vi "Initialize JSON DAO.vi"(10 "Item Name":string="PA Order Tracker", 11 "DB Sufix":string) -> (0 "error out":errorcluster, 3 "Customer DAO JSON out":refnum<class "Object DAO JSON.lvclass">)   [LabVIEW 2020, in "Object DAO JSON.lvclass"]
uses:
  Object DAO JSON.lvclass
  C:/Users/fflores/Desktop/DataBase - Copy - Copy - Copy/Object DAO/Object DAO.lvclass
  Object DAO/Object DAO.lvclass/Object DAO.ctl
  Object DAO JSON.lvclass/Object DAO JSON.ctl
  Object DAO/Member Accessors/Get Item Name.vi
  External Libraries/JSON File Manipulation.lvlibp
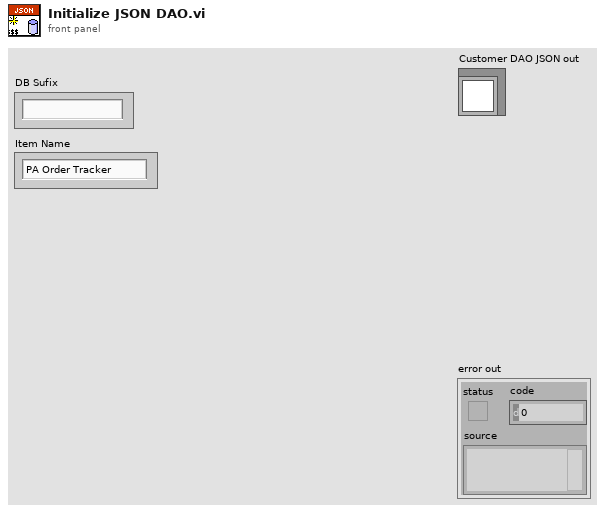
[diagram p1: front panel]
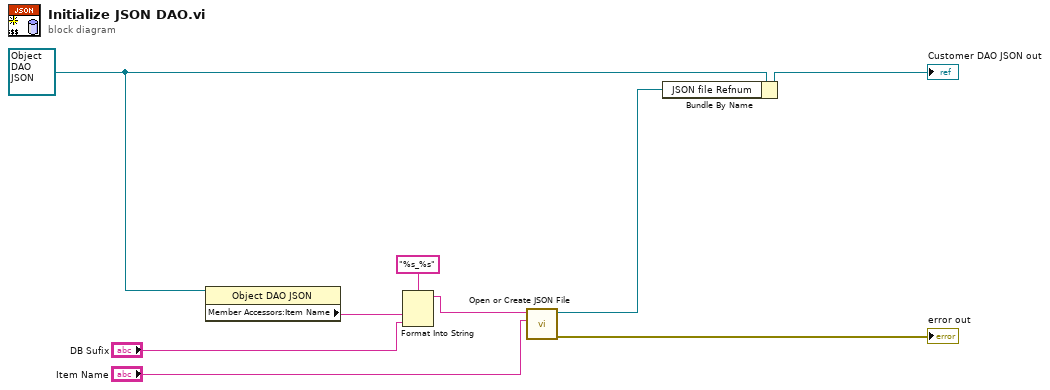
[diagram p0: block diagram]
diagram:
  w6 = refnum<class "Object DAO JSON.lvclass"> refnum ("Customer DAO JSON in")
  n1 = property class="Object DAO JSON"(reference=w6) -> ("Member Accessors:Item Name"=w5:string)  [unwired: 1 in, 2 out]
  n2 = Format Into String(format string="%s_%s", w5, "DB Sufix") -> (resulting string=w2:string)  [unwired: 2 in, 1 out]
  n3 = call "Open or Create JSON File.vi"("Application Name"="Item Name", "Item Name"=w2) -> ("error out"=→"error out":errorcluster, "JSON File Refnum"=w7:refnum<file>)  [unwired: 8 in]
  n4 = Bundle By Name(cluster=w6, "JSON file Refnum"=w7) -> (→"Customer DAO JSON out":refnum<class "Object DAO JSON.lvclass">)
